vi "LINX UART Write Benchmark.vi"() -> ()   [LabVIEW 2013]
uses:
  <vilib>/ptbypt/NI_PtbyPt.lvlib
  <vilib>/LabVIEW Hacker/LINX/LVH-LINX.lvlib
panel:
  out "concatenated string":string
  in  "Stop Button":bool
  out "Loop Rate":dbl(graph)
  out "Loop Time (ms)":i32
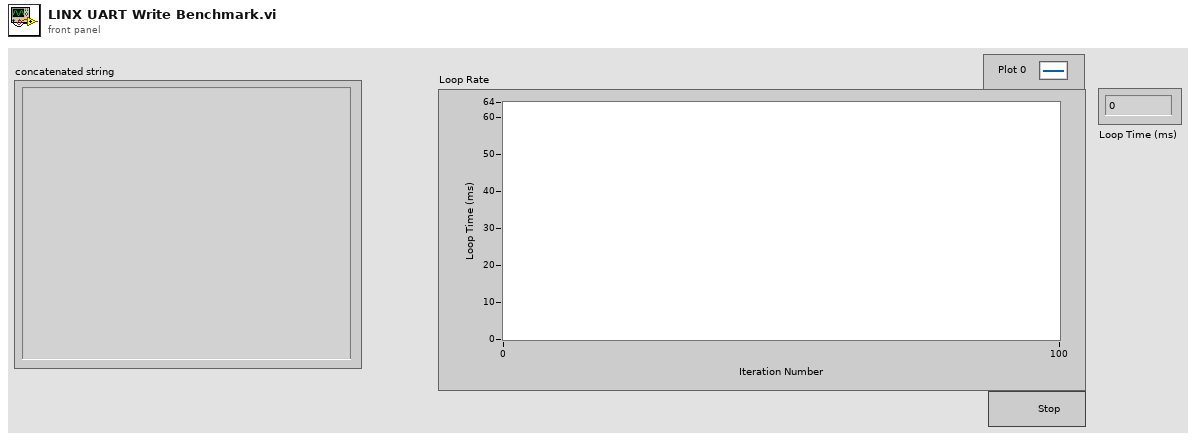
[diagram p1: front panel]
types:
  T1 = typedef "LVH-LINX.lvlib/LINX Ref.ctl" = cluster{"Platform":T2, "Interface":T3, "LINX Device Config":T4}
  T2 = typedef "LVH-LINX.lvlib/Platform.ctl" = enum16{"LINX", "myRIO"}
  T3 = typedef "LVH-LINX.lvlib/Interface.ctl" = enum16{"Serial", "TCP"}
  T4 = typedef "LVH-LINX.lvlib/Device.lvlib/LINX Device Config.ctl" = cluster{"Interface":T3, "COM Port":refnum<visa-resource-name>, "TCP Configuration":T5, "Device Family":T6, "Device ID":u8, "Device Name":string, "TCP Ref":refnum<k5>}
  T5 = typedef "LVH-LINX.lvlib/Device.lvlib/TCP Config.ctl" = cluster{"IP Address":string, "Port":u16}
  T6 = typedef "LVH-LINX.lvlib/Device Family.ctl" = enum8{"National Instruments", "Digilent", "Arduino"}
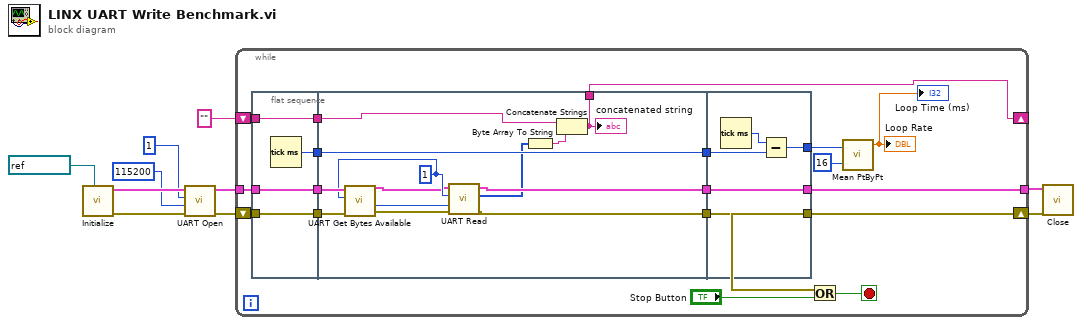
[diagram p0: block diagram]
diagram:
  n1 = call <vilib>:"Initialize.vi"("Serial Port"=refnum<visa-resource-name> "COM5" ("COM Port")) -> ("Error Out"=w8:errorcluster, "LINX Ref"=w9:T1)  [unwired: 8 in, 1 out]
  n2 = call <vilib>:"UART Open.vi"("Error In"=w8, "Baud Rate (9600)"=u32 115200, "UART Channel (0)"=u8 1 ("UART Channel"), "LINX Resource"=w9) -> ("Error Out"=w6:errorcluster, "LINX Resource"=w7:T1)  [unwired: 6 in]
  n3 = while {
    shift-right: [w14] -> w3
    shift-left: w6 -> [w21]
    tunnel: w7 -> [w17]
    tunnel: [w16] -> w2
    shift-right: [w11] -> _
    shift-left: "" ("Data") -> [w12]
    stop <- w28 stop-if-true
    n4 = flat-sequence {
      tunnel: [w32] -> w26
      tunnel: w21 -> [w31]
      tunnel: [w31] -> w20
      tunnel: [w30] -> w18
      tunnel: w17 -> [w30]
      tunnel: [w29] -> w13
      tunnel: w12 -> [w29]
      tunnel: w26 -> [w45]
      tunnel: [w45] -> w25
      tunnel: w20 -> [w41]
      tunnel: [w43] -> w19
      tunnel: w18 -> [w42]
      tunnel: [w44] -> w15
      tunnel: w13 -> [w38]
      tunnel: [w33] -> w11
      tunnel: w25 -> [w49]
      tunnel: [w48] -> w24
      tunnel: [w47] -> w14
      tunnel: w19 -> [w47]
      tunnel: [w46] -> w16
      tunnel: w15 -> [w46]
      frame #0 {
        n5 = Tick Count (ms)() -> (millisecond timer value=w32:u32)
      }
      frame #1 {
        w40 = u8 1 ("UART Channel")
        n6 = call <vilib>:"UART Get Bytes Available.vi"("Error In"=w41, "UART Channel (0)"=w40, "LINX Resource"=w42) -> ("Error Out"=w35:errorcluster, "Bytes Available"=w34:u32, "LINX Resource"=w39:T1)  [unwired: 6 in]
        n7 = call <vilib>:"UART Read.vi"("Error In"=w35, "Num Bytes"=w34, "UART Channel (0)"=w40, "LINX Resource"=w39) -> ("Error Out"=w43:errorcluster, "Data"=w36:u8[], "LINX Resource"=w44:T1)  [unwired: 5 in]
        n8 = Byte Array To String(unsigned byte array=w36) -> (string=w37:string)
        n9 = Concatenate Strings(w38, w37) -> (w33:string)
        "concatenated string" <- w33
      }
      frame #2 {
        n10 = Tick Count (ms)() -> (millisecond timer value=w50:u32)
        n11 = Subtract(x=w50, y=w49) -> (x-y=w48:u32)
      }
    }
    n12 = Or(x=w14, y="Stop Button") -> (x .or. y?=w28:bool)
    n13 = call <vilib>:"Mean PtByPt.vi"("x"=w24, "sample length"=16) -> ("mean"=→"Loop Rate" →"Loop Time (ms)":dbl)  [unwired: 2 in, 1 out]
  }
  n14 = call <vilib>:"Close.vi"("Error In"=w3, "LINX Resource"=w2) -> ()  [unwired: 8 in, 2 out]
